vi "Load_Etch_Cell_Data.vi"() -> (0 "Etch Cell Data":T1)   [LabVIEW 2020]
uses:
  <vilib>/Utility/file.llb/Read Delimited Spreadsheet (string).vi
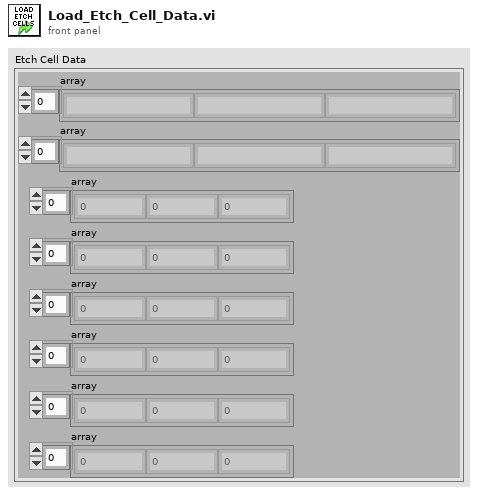
[diagram p1: front panel]
types:
  T1 = cluster{"array":string[], "array":string[], "array":dbl[], "array":dbl[], "array":u32[], "array":u32[], "array":dbl[], "array":i32[]}
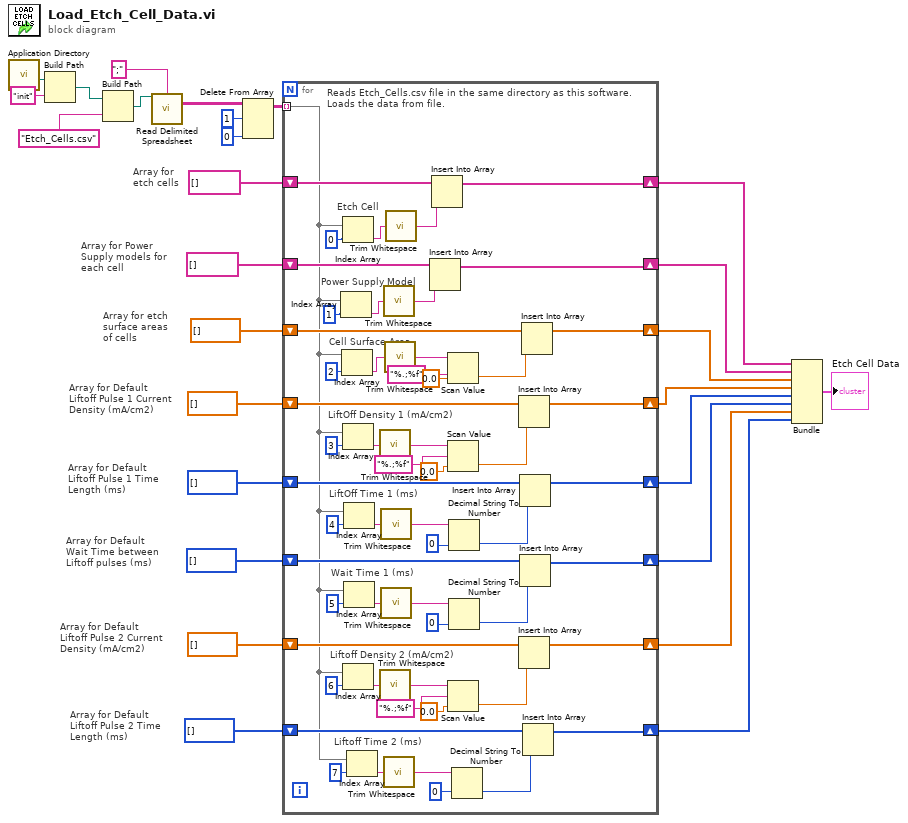
[diagram p0: block diagram]
diagram:
  # "Array for Power \nSupply models for\neach cell"
  # "Array for Default \nLiftoff Pulse 2 Time\nLength (ms)"
  # "Array for Default \nLiftoff Pulse 2 Current\nDensity (mA/cm2)"
  # "Array for Default \nWait Time between\nLiftoff pulses (ms)"
  # "Array for Default \nLiftoff Pulse 1 Time\nLength (ms)"
  # "Array for \netch cells"
  # "Array for Default \nLiftoff Pulse 1 Current\nDensity (mA/cm2)"
  # "Array for etch\nsurface areas\nof cells"
  n1 = call <vilib>:"Application Directory.vi"() -> ("Application Directory"=w2:path)
  n2 = Build Path(base path=w2, name or relative path="init") -> (appended path=w3:path)
  n3 = Build Path(base path=w3, name or relative path="Etch_Cells.csv") -> (appended path=w27:path)
  n4 = call-poly <vilib>:"Read Delimited Spreadsheet.vi"("file path (dialog if empty)"=w27, "delimiter (\\t)"=";" ("delimiter (\\t)")) -> ("all rows"=w26:string[][])  [unwired: 8 in, 5 out]
  n5 = Delete From Array(array=w26, length=1, index (row)=0) -> (array with subset deleted=w23:string[][])  [unwired: 1 in, 1 out]
  n6 = for {
    tunnel: w23 -> [w28] mode=indexing
    shift-right: [w76] -> w13
    shift-left: dbl[] [] ("array") -> [w77]
    shift-right: [w73] -> w9
    shift-left: dbl[] [] ("array") -> [w74]
    shift-right: [w68] -> w12
    shift-left: string[] [] ("array") -> [w69]
    shift-right: [w58] -> w8
    shift-left: u32[] [] ("array") -> [w59]
    shift-right: [w51] -> w7
    shift-left: u32[] [] ("array") -> [w52]
    shift-right: [w44] -> w6
    shift-left: dbl[] [] ("array") -> [w45]
    shift-right: [w38] -> w5
    shift-left: i32[] [] ("array") -> [w39]
    shift-right: [w29] -> w10
    shift-left: string[] [] ("array") -> [w30]
    # "Power Supply Model"
    # "Liftoff Time 2 (ms)"
    # "Liftoff Density 2 (mA/cm2)"
    # "Wait Time 1 (ms)"
    # "LiftOff Time 1 (ms)"
    # "Reads Etch_Cells.csv file in the same directory as this software.\nLoads the data from file."
    # "Etch Cell"
    # "LiftOff Density 1 (mA/cm2)"
    # "Cell Surface Area"
    n7 = Index Array(array=w28, index=1) -> (element=w32:string)
    n8 = Index Array(array=w28, index=2) -> (element=w81:string)
    n9 = Index Array(array=w28, index=0) -> (element=w71:string)
    n10 = Index Array(array=w28, index=3) -> (element=w80:string)
    n11 = Index Array(array=w28, index=6) -> (element=w49:string)
    n12 = Index Array(array=w28, index=4) -> (element=w63:string)
    n13 = Index Array(array=w28, index=5) -> (element=w56:string)
    n14 = Index Array(array=w28, index=7) -> (element=w42:string)
    n15 = call <vilib>:"Trim Whitespace.vi"("string"=w80) -> ("trimmed string"=w79:string)  [unwired: 1 in]
    n16 = call <vilib>:"Trim Whitespace.vi"("string"=w49) -> ("trimmed string"=w48:string)  [unwired: 1 in]
    n17 = call <vilib>:"Trim Whitespace.vi"("string"=w63) -> ("trimmed string"=w62:string)  [unwired: 1 in]
    n18 = call <vilib>:"Trim Whitespace.vi"("string"=w56) -> ("trimmed string"=w55:string)  [unwired: 1 in]
    n19 = call <vilib>:"Trim Whitespace.vi"("string"=w32) -> ("trimmed string"=w31:string)  [unwired: 1 in]
    n20 = call <vilib>:"Trim Whitespace.vi"("string"=w42) -> ("trimmed string"=w41:string)  [unwired: 1 in]
    n21 = call <vilib>:"Trim Whitespace.vi"("string"=w81) -> ("trimmed string"=w66:string)  [unwired: 1 in]
    n22 = call <vilib>:"Trim Whitespace.vi"("string"=w71) -> ("trimmed string"=w70:string)  [unwired: 1 in]
    n23 = Insert Into Array(array=w30, new element=w31) -> (w29:string[])  [unwired: 1 in]
    n24 = Insert Into Array(array=w69, new element=w70) -> (w68:string[])  [unwired: 1 in]
    n25 = Scan Value(string=w66, format string="%.;%f", default (0 dbl)=0.0) -> (value=w65:dbl)  [unwired: 1 out]
    n26 = Scan Value(string=w79, format string="%.;%f", default (0 dbl)=0.0) -> (value=w75:dbl)  [unwired: 1 out]
    n27 = Scan Value(string=w48, format string="%.;%f", default (0 dbl)=0.0) -> (value=w46:dbl)  [unwired: 1 out]
    n28 = Decimal String To Number(string=w62, default (0L)=u32 0) -> (number=w60:u32)  [unwired: 1 in, 1 out]
    n29 = Decimal String To Number(string=w55, default (0L)=u32 0) -> (number=w53:u32)  [unwired: 1 in, 1 out]
    n30 = Decimal String To Number(string=w41, default (0L)=u32 0) -> (number=w40:u32)  [unwired: 1 in, 1 out]
    n31 = Insert Into Array(array=w74, new element=w75) -> (w73:dbl[])  [unwired: 1 in]
    n32 = Insert Into Array(array=w45, new element=w46) -> (w44:dbl[])  [unwired: 1 in]
    n33 = Insert Into Array(array=w59, new element=w60) -> (w58:u32[])  [unwired: 1 in]
    n34 = Insert Into Array(array=w52, new element=w53) -> (w51:u32[])  [unwired: 1 in]
    n35 = Insert Into Array(array=w77, new element=w65) -> (w76:dbl[])  [unwired: 1 in]
    n36 = Insert Into Array(array=w39, new element=w40) -> (w38:i32[])  [unwired: 1 in]
  }
  n37 = Bundle("array"=w12, "array"=w10, "array"=w13, "array"=w9, "array"=w8, "array"=w7, "array"=w6, "array"=w5) -> (→"Etch Cell Data":T1)  [unwired: 1 in]
